vi "stop.vi"(8 "error in (no error)":errorcluster, 11 "FPGA in":refnum<class "FPGA.lvclass">) -> (0 "error out":errorcluster, 3 "FPGA out":refnum<class "FPGA.lvclass">)   [LabVIEW 2016, in "FPGA.lvclass"]
uses:
  FPGA.lvclass
  FPGA.lvclass/FPGA.ctl
  <vilib>/FPGAPlugInAG/Dynamic/niLvFpga_Abort_Dynamic.vi
  <vilib>/FPGAPlugInAG/Dynamic/niLvFpga_Close_Dynamic.vi
  <vilib>/rvi/interface/nirviMethod/nirviMethod.xnode
  <vilib>/rvi/interface/nirviCloseFPGA/nirviCloseFPGA.xnode
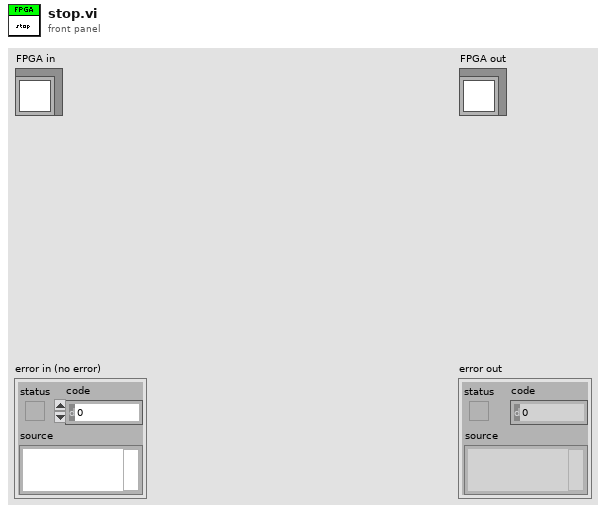
[diagram p1: front panel]
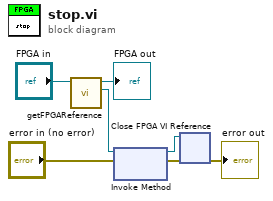
[diagram p0: block diagram]
diagram:
  n1 = call "getFPGAReference.vi"("FPGA in"="FPGA in") -> ("FPGAReference"=w6:refnum<k20>, "FPGA out"=→"FPGA out":refnum<class "FPGA.lvclass">)  [unwired: 9 in]
  n2 = xnode "Invoke Method"("FPGA VI Reference In"=w6, "error in"="error in (no error)") -> ("FPGA VI Reference Out"=w5:refnum<k20>, "error out"=w4:errorcluster)
  n3 = xnode "Close FPGA VI Reference"("FPGA VI Reference In"=w5, "error in"=w4) -> ("error out"=→"error out":errorcluster)
